vi "amplitude Spectrum from DAQ cernox removed.vi"(11 "Sample Duration (sec)":u32(knob)=31 scale=1.0..33.0) -> ()   [LabVIEW 2010]
uses:
  <vilib>/Analysis/2dsp.llb/Complex FFT.vi
  <vilib>/Analysis/NI_AALPro.lvlib
panel:
  out "error out":errorcluster
  out "Numeric":dbl=1484646840.0
  out "size(s)":i32=257
  out "Temp (K)":dbl=285.2027629999985 format="%_5g"
  in  "?":u16(ring)=5 items=["2", "4", "8", "16", "32", "64", "128", "256", "512", "8192", "1024", "2048", "4096", "8192", "16384", "32768", "65536", "131072", "262144", "524288 (one Channel)"]
  out "Spring Constant":dbl=0.016711730050282706
  out "<X^2>":dbl=2.3562204125555914e-19
  in  "Vpp":dbl=2.0
  out "x/y":cdb[](array[numeric])=[1.822835740797244e-23+0.0i, 1.7675640290457217e-23+0.0i, 1.4131702570700112e-23+0.0i, 2.223228937284431e-23+0.0i, 1.8861746568658304e-23+0.0i, 1.7224162597684228e-23+0.0i, 1.9293974775985452e-23+0.0i, 1.7742568740748702e-23+0.0i, 1.7769988182972965e-23+0.0i, 1.696176827526328e-23+0.0i, 1.8264193162076468e-23+0.0i, 1.9320144282170158e-23+0.0i, 2.0438742275850636e-23+0.0i, 2.222965311780456e-23+0.0i, 2.2549713226001863e-23+0.0i, 1.768885151694379e-23+0.0i, 2.176124999620469e-23+0.0i, 2.129234808266423e-23+0.0i, 2.067533774251591e-23+0.0i, 2.8427194668312566e-23+0.0i, 4.7553300725519583e-23+0.0i, 7.584325194857353e-23+0.0i, 2.1639134957441051e-23+0.0i, 2.5848083814905796e-23+0.0i, 2.851360155046589e-23+0.0i, 2.800634573630391e-23+0.0i, 2.338011797798725e-23+0.0i, 1.765079942656028e-23+0.0i, 2.104025187275973e-23+0.0i, 2.388051905691794e-23+0.0i, 2.853642619630031e-23+0.0i, 2.6711089516925724e-23+0.0i, 3.0459849796946806e-23+0.0i, 2.4401708416353815e-23+0.0i, 2.680531554902485e-23+0.0i, 2.9187825564451e-23+0.0i, 2.757565093207759e-23+0.0i, 3.035983267786727e-23+0.0i, 3.0910445814793146e-23+0.0i, 2.6051056874131243e-23+0.0i, 3.3956681306471256e-23+0.0i, 1.440691698306415e-22+0.0i, 6.100033131698352e-23+0.0i, 4.785561997662565e-23+0.0i, 4.4124379844200306e-23+0.0i, 4.1259461883143996e-23+0.0i, 3.976691477576303e-23+0.0i, 3.3602145359711534e-23+0.0i, 4.0934370310497964e-23+0.0i, 3.5625122285956665e-23+0.0i, 4.741274194370224e-23+0.0i, 4.622208059213624e-23+0.0i, 3.9223525205613755e-23+0.0i, 5.48665968324749e-23+0.0i, 3.875217807549581e-23+0.0i, 4.7796852328905696e-23+0.0i, 4.186904482333236e-23+0.0i, 6.049046606211197e-23+0.0i, 4.7905740078949955e-23+0.0i, 5.966921181453847e-23+0.0i, 5.130685417892801e-23+0.0i, 6.447729060239504e-23+0.0i, 6.070995523877117e-23+0.0i, 6.695912635778031e-23+0.0i, 5.982200688789285e-23+0.0i, 6.953655879559275e-23+0.0i, 7.719151718181244e-23+0.0i, 6.283551098164771e-23+0.0i, 6.616623115972441e-23+0.0i, 7.596763060682753e-23+0.0i, 7.333888292538558e-23+0.0i, 8.555537111075796e-23+0.0i, 9.5817232840548e-23+0.0i, 1.3181714014662204e-22+0.0i, 9.157484291226144e-23+0.0i, 7.751487205370229e-23+0.0i, 9.705897696242533e-23+0.0i, 1.0223323442116599e-22+0.0i, 1.0459001593217017e-22+0.0i, 1.1453450352921381e-22+0.0i, 1.2931657458720736e-22+0.0i, 1.459314628472842e-22+0.0i, 1.4070158876888328e-22+0.0i, 1.2605113149888989e-22+0.0i, 1.509819076598123e-22+0.0i, 1.544803841468646e-22+0.0i, 1.7700865059628094e-22+0.0i, 1.5376972478878197e-22+0.0i, 1.774728514817178e-22+0.0i, 1.8428914385759788e-22+0.0i, 2.2701171686531848e-22+0.0i, 1.838974511711876e-22+0.0i, 2.3627238680060907e-22+0.0i, 2.6269788328421313e-22+0.0i, 3.1051675808314644e-22+0.0i, 3.1120553407649953e-22+0.0i, 2.474307852966178e-22+0.0i, 3.341689824691674e-22+0.0i, 3.4471645453619096e-22+0.0i, 3.893320019912561e-22+0.0i, 4.1555515373755697e-22+0.0i, 5.455595521720538e-22+0.0i, 4.19934391425876e-22+0.0i, 4.908920977628759e-22+0.0i, 6.54725607731936e-22+0.0i, 5.404398330184923e-22+0.0i, 5.070609745440634e-22+0.0i, 7.501899902695688e-22+0.0i, 7.690047558843619e-22+0.0i, 8.091732940709215e-22+0.0i, 1.3031158912345799e-21+0.0i, 1.1512072647056174e-21+0.0i, 1.5268653969019806e-21+0.0i, 1.2878353575945014e-21+0.0i, 1.5861964752201703e-21+0.0i, 2.0874276416653818e-21+0.0i, 2.1537295587433287e-21+0.0i, 2.609801356487359e-21+0.0i, 2.794904862045169e-21+0.0i, 4.450890917281775e-21+0.0i, 4.782323183717228e-21+0.0i, 7.332879493133011e-21+0.0i, 8.720096388166533e-21+0.0i, 1.2048295246993849e-20+0.0i, 1.2445896073270755e-20+0.0i, 1.621889890374649e-20+0.0i, 2.5789862100239256e-20+0.0i, 1.7162750008545038e-20+0.0i, 1.6981422368097548e-20+0.0i, 1.1590736557342194e-20+0.0i, 9.14433437194095e-21+0.0i, 8.479983483390395e-21+0.0i, 6.568566536262503e-21+0.0i, 5.68343630205877e-21+0.0i, 4.478108035357037e-21+0.0i, 3.3395244446396683e-21+0.0i, 2.7493880233410565e-21+0.0i, 2.8389909650442048e-21+0.0i, 2.10455365672315e-21+0.0i, 1.5813034454830923e-21+0.0i, 1.2930365806113183e-21+0.0i, 1.2472170782254345e-21+0.0i, 1.1031647973872676e-21+0.0i, 8.8935516799099e-22+0.0i, 8.813468505072157e-22+0.0i, 8.834919269545325e-22+0.0i, 7.189279924592954e-22+0.0i, 8.018325795498779e-22+0.0i, 6.887070160521788e-22+0.0i, 7.329693497748081e-22+0.0i, 1.0058798260443032e-21+0.0i, 9.647467233858385e-22+0.0i, 5.881439114977712e-22+0.0i, 4.749433371668375e-22+0.0i, 3.6445918034601733e-22+0.0i, 2.8553400941847603e-22+0.0i, 3.9590897313916664e-22+0.0i, 3.3470734663309492e-22+0.0i, 3.2677511578285326e-22+0.0i, 2.7568964497043927e-22+0.0i, 2.243714895267099e-22+0.0i, 2.3930849601002674e-22+0.0i, 2.1787404973653707e-22+0.0i, 2.564842365349928e-22+0.0i, 1.8072546820279964e-22+0.0i, 2.008643480727801e-22+0.0i, 2.0432481222384193e-22+0.0i, 1.5072645039398344e-22+0.0i, 1.1578159171670506e-22+0.0i, 1.3856476941890455e-22+0.0i, 1.5750834082476817e-22+0.0i, 1.6598137898047965e-22+0.0i, 1.6846717057439265e-22+0.0i, 1.0637472542076113e-22+0.0i, 1.204765852625695e-22+0.0i, 1.1192400535353832e-22+0.0i, 9.586293087531511e-23+0.0i, 1.05741985863128e-22+0.0i, 1.0756461776754148e-22+0.0i, 1.0633342834367033e-22+0.0i, 9.41450875281874e-23+0.0i, 9.796297730479969e-23+0.0i, 8.991253125127156e-23+0.0i, 7.21495012420243e-23+0.0i, 8.108566724947074e-23+0.0i, 8.065267752833244e-23+0.0i, 8.159100620339912e-23+0.0i, 6.537407040699658e-23+0.0i, 6.065196292025972e-23+0.0i, 6.912565683967239e-23+0.0i, 4.585047711312349e-23+0.0i, 5.407319623212663e-23+0.0i, 5.662637982484711e-23+0.0i, 6.826102675920094e-23+0.0i, 5.317752314345768e-23+0.0i, 6.080938507048622e-23+0.0i, 5.580121915088842e-23+0.0i, 5.08599202552338e-23+0.0i, 5.757992131668778e-23+0.0i, 5.06295037704728e-23+0.0i, 4.0664759451789855e-23+0.0i, 8.778521018866551e-23+0.0i, 7.277091477651407e-23+0.0i, 3.968581632591024e-23+0.0i, 4.7007347174208957e-23+0.0i, 3.794186298189703e-23+0.0i, 4.820976496823016e-23+0.0i, 3.601765577546427e-23+0.0i, 3.459047542602718e-23+0.0i, 2.922903524340481e-23+0.0i, 3.570082548445812e-23+0.0i, 4.2755954972988234e-23+0.0i, 6.38478352818444e-23+0.0i, 1.601945502273552e-22+0.0i, 4.1400733672163123e-23+0.0i, 3.208702560959063e-23+0.0i, 3.3199369569753925e-23+0.0i, 2.7585085524308984e-23+0.0i, 3.131294045384947e-23+0.0i, 3.132076096760791e-23+0.0i, 2.5044550632070505e-23+0.0i, 2.996800434607099e-23+0.0i, 2.603310734333486e-23+0.0i, 2.3624545316458745e-23+0.0i, 2.8416716343560486e-23+0.0i, 2.5713096089926784e-23+0.0i, 2.3991585444755748e-23+0.0i, 2.3758300262426874e-23+0.0i, 2.894242043071023e-23+0.0i, 3.0079952252920497e-23+0.0i, 2.687090320067224e-23+0.0i, 3.060055893657326e-23+0.0i, 2.588927969919409e-23+0.0i, 1.3050755525240973e-22+0.0i, 6.369169567192907e-23+0.0i, 2.768674461007611e-23+0.0i, 1.996611478830249e-23+0.0i, 2.2847349020279004e-23+0.0i, 2.178447279898464e-23+0.0i, 1.611552403721389e-23+0.0i, 2.238567254293866e-23+0.0i, 2.0453257588723553e-23+0.0i, 2.2271941970345648e-23+0.0i, 2.0056331268074712e-23+0.0i, 1.60966633920541e-23+0.0i, 1.6230214465249225e-23+0.0i, 2.0086198141015995e-23+0.0i, 2.011029187025087e-23+0.0i, 1.980316992576717e-23+0.0i, 1.882256216302402e-23+0.0i, 1.974131492412098e-23+0.0i, 2.326555234354055e-23+0.0i, 1.515444684592899e-23+0.0i, 1.6225332592048996e-23+0.0i, 1.8662819972339634e-23+0.0i, 2.3769145357012108e-23+0.0i]
  out "df (Hz)":dbl=0.125
  out "time intervals":dbl=4.0
  out "iterations":dbl=64.0
  in  "# of points to collect":u16(ring)=2 items=["64", "128", "256", "512", "1024", "2048", "4096", "8192", "16384", "32768", "65536", "131072", "262144", "524288"]
  out "Cycles":dbl=1.0
  in  "Averages":dbl=1.0
  out "Total  points":dbl=16384.0
  out "XY Graph 3":cluster{dbl, dbl}[](graph)=[{6354.705, 1.822835740797244e-23}, {6354.83, 1.7675640290457217e-23}, {6354.955, 1.4131702570700112e-23}, {6355.08, 2.223228937284431e-23}, {6355.205, 1.8861746568658304e-23}, {6355.33, 1.7224162597684228e-23}, {6355.455, 1.9293974775985452e-23}, {6355.58, 1.7742568740748702e-23}, {6355.705, 1.7769988182972965e-23}, {6355.83, 1.696176827526328e-23}, {6355.955, 1.8264193162076468e-23}, {6356.08, 1.9320144282170158e-23}, {6356.205, 2.0438742275850636e-23}, {6356.33, 2.222965311780456e-23}, {6356.455, 2.2549713226001863e-23}, {6356.58, 1.768885151694379e-23}, {6356.705, 2.176124999620469e-23}, {6356.83, 2.129234808266423e-23}, {6356.955, 2.067533774251591e-23}, {6357.08, 2.8427194668312566e-23}, {6357.205, 4.7553300725519583e-23}, {6357.33, 7.584325194857353e-23}, {6357.455, 2.1639134957441051e-23}, {6357.58, 2.5848083814905796e-23}, {6357.705, 2.851360155046589e-23}, {6357.83, 2.800634573630391e-23}, {6357.955, 2.338011797798725e-23}, {6358.08, 1.765079942656028e-23}, {6358.205, 2.104025187275973e-23}, {6358.33, 2.388051905691794e-23}, {6358.455, 2.853642619630031e-23}, {6358.58, 2.6711089516925724e-23}, {6358.705, 3.0459849796946806e-23}, {6358.83, 2.4401708416353815e-23}, {6358.955, 2.680531554902485e-23}, {6359.08, 2.9187825564451e-23}, {6359.205, 2.757565093207759e-23}, {6359.33, 3.035983267786727e-23}, {6359.455, 3.0910445814793146e-23}, {6359.58, 2.6051056874131243e-23}, {6359.705, 3.3956681306471256e-23}, {6359.83, 1.440691698306415e-22}, {6359.955, 6.100033131698352e-23}, {6360.08, 4.785561997662565e-23}, {6360.205, 4.4124379844200306e-23}, {6360.33, 4.1259461883143996e-23}, {6360.455, 3.976691477576303e-23}, {6360.58, 3.3602145359711534e-23}, {6360.705, 4.0934370310497964e-23}, {6360.83, 3.5625122285956665e-23}, {6360.955, 4.741274194370224e-23}, {6361.08, 4.622208059213624e-23}, {6361.205, 3.9223525205613755e-23}, {6361.33, 5.48665968324749e-23}, {6361.455, 3.875217807549581e-23}, {6361.58, 4.7796852328905696e-23}, {6361.705, 4.186904482333236e-23}, {6361.83, 6.049046606211197e-23}, {6361.955, 4.7905740078949955e-23}, {6362.08, 5.966921181453847e-23}, {6362.205, 5.130685417892801e-23}, {6362.33, 6.447729060239504e-23}, {6362.455, 6.070995523877117e-23}, {6362.58, 6.695912635778031e-23}, {6362.705, 5.982200688789285e-23}, {6362.83, 6.953655879559275e-23}, {6362.955, 7.719151718181244e-23}, {6363.08, 6.283551098164771e-23}, {6363.205, 6.616623115972441e-23}, {6363.33, 7.596763060682753e-23}, {6363.455, 7.333888292538558e-23}, {6363.58, 8.555537111075796e-23}, {6363.705, 9.5817232840548e-23}, {6363.83, 1.3181714014662204e-22}, {6363.955, 9.157484291226144e-23}, {6364.08, 7.751487205370229e-23}, {6364.205, 9.705897696242533e-23}, {6364.33, 1.0223323442116599e-22}, {6364.455, 1.0459001593217017e-22}, {6364.58, 1.1453450352921381e-22}, {6364.705, 1.2931657458720736e-22}, {6364.83, 1.459314628472842e-22}, {6364.955, 1.4070158876888328e-22}, {6365.08, 1.2605113149888989e-22}, {6365.205, 1.509819076598123e-22}, {6365.33, 1.544803841468646e-22}, {6365.455, 1.7700865059628094e-22}, {6365.58, 1.5376972478878197e-22}, {6365.705, 1.774728514817178e-22}, {6365.83, 1.8428914385759788e-22}, {6365.955, 2.2701171686531848e-22}, {6366.08, 1.838974511711876e-22}, {6366.205, 2.3627238680060907e-22}, {6366.33, 2.6269788328421313e-22}, {6366.455, 3.1051675808314644e-22}, {6366.58, 3.1120553407649953e-22}, {6366.705, 2.474307852966178e-22}, {6366.83, 3.341689824691674e-22}, {6366.955, 3.4471645453619096e-22}, {6367.08, 3.893320019912561e-22}, {6367.205, 4.1555515373755697e-22}, {6367.33, 5.455595521720538e-22}, {6367.455, 4.19934391425876e-22}, {6367.58, 4.908920977628759e-22}, {6367.705, 6.54725607731936e-22}, {6367.83, 5.404398330184923e-22}, {6367.955, 5.070609745440634e-22}, {6368.08, 7.501899902695688e-22}, {6368.205, 7.690047558843619e-22}, {6368.33, 8.091732940709215e-22}, {6368.455, 1.3031158912345799e-21}, {6368.58, 1.1512072647056174e-21}, {6368.705, 1.5268653969019806e-21}, {6368.83, 1.2878353575945014e-21}, {6368.955, 1.5861964752201703e-21}, {6369.08, 2.0874276416653818e-21}, {6369.205, 2.1537295587433287e-21}, {6369.33, 2.609801356487359e-21}, {6369.455, 2.794904862045169e-21}, {6369.58, 4.450890917281775e-21}, {6369.705, 4.782323183717228e-21}, {6369.83, 7.332879493133011e-21}, {6369.955, 8.720096388166533e-21}, {6370.08, 1.2048295246993849e-20}, {6370.205, 1.2445896073270755e-20}, {6370.33, 1.621889890374649e-20}, {6370.455, 2.5789862100239256e-20}, {6370.58, 1.7162750008545038e-20}, {6370.705, 1.6981422368097548e-20}, {6370.83, 1.1590736557342194e-20}, {6370.955, 9.14433437194095e-21}, {6371.08, 8.479983483390395e-21}, {6371.205, 6.568566536262503e-21}, {6371.33, 5.68343630205877e-21}, {6371.455, 4.478108035357037e-21}, {6371.58, 3.3395244446396683e-21}, {6371.705, 2.7493880233410565e-21}, {6371.83, 2.8389909650442048e-21}, {6371.955, 2.10455365672315e-21}, {6372.08, 1.5813034454830923e-21}, {6372.205, 1.2930365806113183e-21}, {6372.33, 1.2472170782254345e-21}, {6372.455, 1.1031647973872676e-21}, {6372.58, 8.8935516799099e-22}, {6372.705, 8.813468505072157e-22}, {6372.83, 8.834919269545325e-22}, {6372.955, 7.189279924592954e-22}, {6373.08, 8.018325795498779e-22}, {6373.205, 6.887070160521788e-22}, {6373.33, 7.329693497748081e-22}, {6373.455, 1.0058798260443032e-21}, {6373.58, 9.647467233858385e-22}, {6373.705, 5.881439114977712e-22}, {6373.83, 4.749433371668375e-22}, {6373.955, 3.6445918034601733e-22}, {6374.08, 2.8553400941847603e-22}, {6374.205, 3.9590897313916664e-22}, {6374.33, 3.3470734663309492e-22}, {6374.455, 3.2677511578285326e-22}, {6374.58, 2.7568964497043927e-22}, {6374.705, 2.243714895267099e-22}, {6374.83, 2.3930849601002674e-22}, {6374.955, 2.1787404973653707e-22}, {6375.08, 2.564842365349928e-22}, {6375.205, 1.8072546820279964e-22}, {6375.33, 2.008643480727801e-22}, {6375.455, 2.0432481222384193e-22}, {6375.58, 1.5072645039398344e-22}, {6375.705, 1.1578159171670506e-22}, {6375.83, 1.3856476941890455e-22}, {6375.955, 1.5750834082476817e-22}, {6376.08, 1.6598137898047965e-22}, {6376.205, 1.6846717057439265e-22}, {6376.33, 1.0637472542076113e-22}, {6376.455, 1.204765852625695e-22}, {6376.58, 1.1192400535353832e-22}, {6376.705, 9.586293087531511e-23}, {6376.83, 1.05741985863128e-22}, {6376.955, 1.0756461776754148e-22}, {6377.08, 1.0633342834367033e-22}, {6377.205, 9.41450875281874e-23}, {6377.33, 9.796297730479969e-23}, {6377.455, 8.991253125127156e-23}, {6377.58, 7.21495012420243e-23}, {6377.705, 8.108566724947074e-23}, {6377.83, 8.065267752833244e-23}, {6377.955, 8.159100620339912e-23}, {6378.08, 6.537407040699658e-23}, {6378.205, 6.065196292025972e-23}, {6378.33, 6.912565683967239e-23}, {6378.455, 4.585047711312349e-23}, {6378.58, 5.407319623212663e-23}, {6378.705, 5.662637982484711e-23}, {6378.83, 6.826102675920094e-23}, {6378.955, 5.317752314345768e-23}, {6379.08, 6.080938507048622e-23}, {6379.205, 5.580121915088842e-23}, {6379.33, 5.08599202552338e-23}, {6379.455, 5.757992131668778e-23}, {6379.58, 5.06295037704728e-23}, {6379.705, 4.0664759451789855e-23}, {6379.83, 8.778521018866551e-23}, {6379.955, 7.277091477651407e-23}, {6380.08, 3.968581632591024e-23}, {6380.205, 4.7007347174208957e-23}, {6380.33, 3.794186298189703e-23}, {6380.455, 4.820976496823016e-23}, {6380.58, 3.601765577546427e-23}, {6380.705, 3.459047542602718e-23}, {6380.83, 2.922903524340481e-23}, {6380.955, 3.570082548445812e-23}, {6381.08, 4.2755954972988234e-23}, {6381.205, 6.38478352818444e-23}, {6381.33, 1.601945502273552e-22}, {6381.455, 4.1400733672163123e-23}, {6381.58, 3.208702560959063e-23}, {6381.705, 3.3199369569753925e-23}, {6381.83, 2.7585085524308984e-23}, {6381.955, 3.131294045384947e-23}, {6382.08, 3.132076096760791e-23}, {6382.205, 2.5044550632070505e-23}, {6382.33, 2.996800434607099e-23}, {6382.455, 2.603310734333486e-23}, {6382.58, 2.3624545316458745e-23}, {6382.705, 2.8416716343560486e-23}, {6382.83, 2.5713096089926784e-23}, {6382.955, 2.3991585444755748e-23}, {6383.08, 2.3758300262426874e-23}, {6383.205, 2.894242043071023e-23}, {6383.33, 3.0079952252920497e-23}, {6383.455, 2.687090320067224e-23}, {6383.58, 3.060055893657326e-23}, {6383.705, 2.588927969919409e-23}, {6383.83, 1.3050755525240973e-22}, {6383.955, 6.369169567192907e-23}, {6384.08, 2.768674461007611e-23}, {6384.205, 1.996611478830249e-23}, {6384.33, 2.2847349020279004e-23}, {6384.455, 2.178447279898464e-23}, {6384.58, 1.611552403721389e-23}, {6384.705, 2.238567254293866e-23}, {6384.83, 2.0453257588723553e-23}, {6384.955, 2.2271941970345648e-23}, {6385.08, 2.0056331268074712e-23}, {6385.205, 1.60966633920541e-23}, {6385.33, 1.6230214465249225e-23}, {6385.455, 2.0086198141015995e-23}, {6385.58, 2.011029187025087e-23}, {6385.705, 1.980316992576717e-23}, {6385.83, 1.882256216302402e-23}, {6385.955, 1.974131492412098e-23}, {6386.08, 2.326555234354055e-23}, {6386.205, 1.515444684592899e-23}, {6386.33, 1.6225332592048996e-23}, {6386.455, 1.8662819972339634e-23}, {6386.58, 2.3769145357012108e-23}]
  out "freq range (hz)":dbl=32.0
  out "dt (s)":dbl=0.015625
  in  "Sensitivity":u16(ring)=22 items=["2 nV/fA", "5 nV/fA", "10 nV/fA", "20 nV/fA", "50 nV/fA", "100 nV/fA", "200 nV/fA", "500 nV/fA", "1 uV/pA", "2 uV/pA", "5 uV/pA", "10 uV/pA", "20 uV/pA", "50 uV/pA", "100 uV/pA", "200 uV/pA", "500 uV/pA", "1 mV/nA", "2 mV/nA", "5 mV/nA", "10 mV/nA", "20 mV/nA", "50 mV/nA", "100 mV/nA", "200 mV/nA", "500 mV/nA", "1 V/uA"]
  in  "Data to Store":u16(ring) items=["X and Y", "R and Theta"]
  in  "Sampling Rate":u16(ring)=13 items=["62.5 mHz", "125 mHz", "250 mHz", "500 mHz", "1 Hz", "2 Hz", "4 Hz", "8 Hz", "16 Hz", "32 Hz", "64 Hz, 256 s wait", "128 Hz, 128 s wait", "256 Hz, 64 s wait", "512 Hz, 32 s wait"]
  in  "Center Frequency [Hz]":dbl=6370.58 format="%.3f"
  in  "Detection Bandwidth":u16(ring)=5 items=["25 kHz", "8.33 kHz", "2.50 kHz", "833 Hz", "250 Hz", "83.3 Hz", "25 Hz", "8.33 Hz", "2.50 Hz", "0.833 Hz", "0.250 Hz", "0.0833 Hz", "0.025 Hz"]
  in  "DS 345 GPIB Address":i32=19
  in  "SR 830 GPIB Address":i32=8
  # "Bandwidth>\n2*samp rate"
  # "SR 830"
  # "Adquisition DAQ"
  # "Sample Rate DAQ"
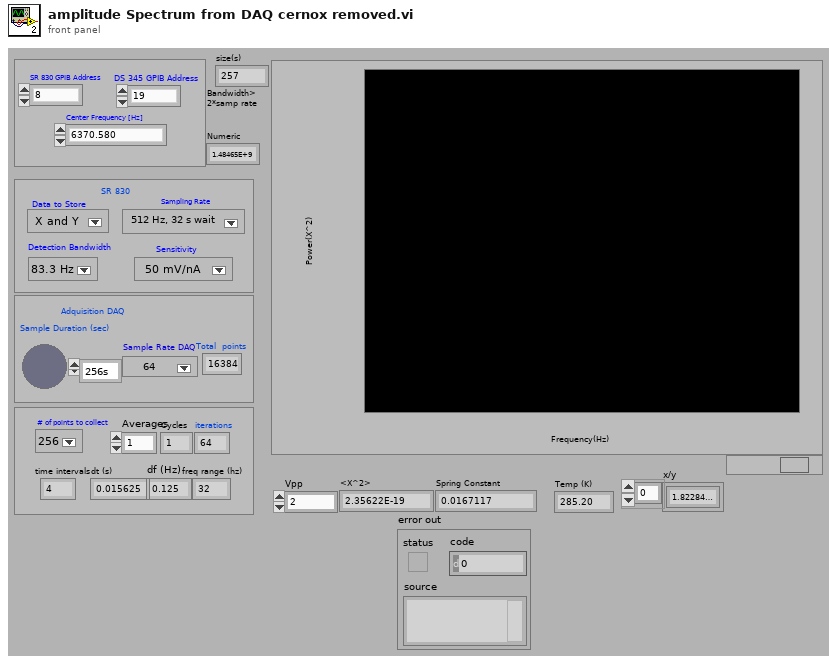
[diagram p1: front panel]
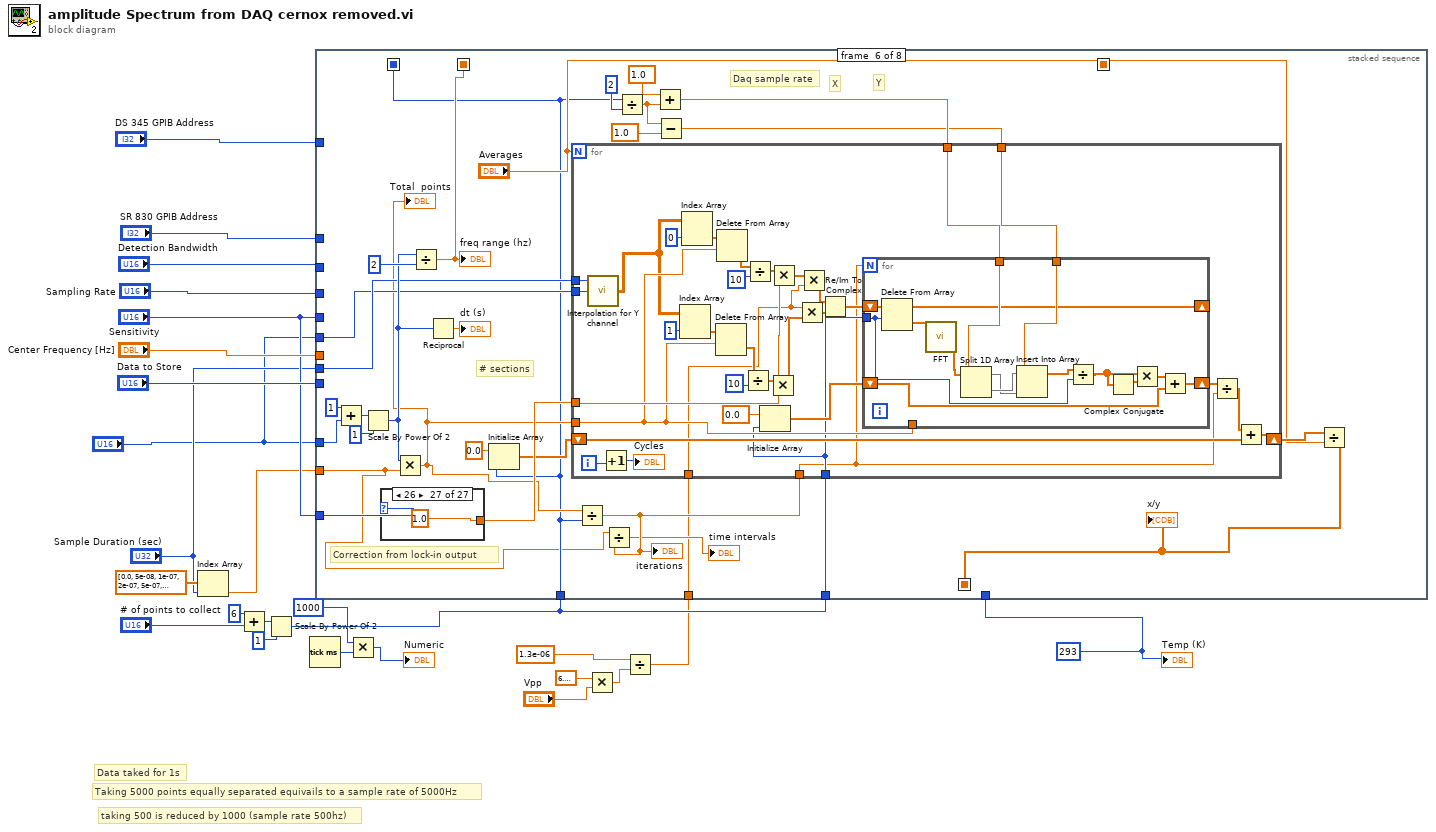
[diagram p0: block diagram]
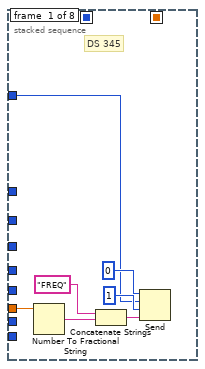
[diagram p2: hidden frame]
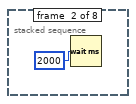
[diagram p3: hidden frame]
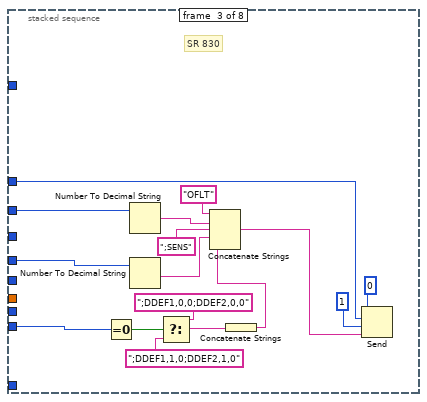
[diagram p4: hidden frame]
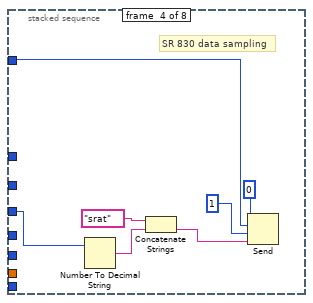
[diagram p5: hidden frame]
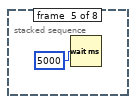
[diagram p6: hidden frame]
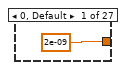
[diagram p7: hidden frame]
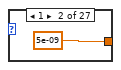
[diagram p8: hidden frame]
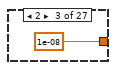
[diagram p9: hidden frame]
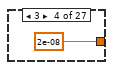
[diagram p10: hidden frame]
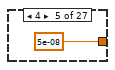
[diagram p11: hidden frame]
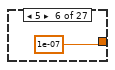
[diagram p12: hidden frame]
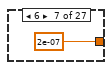
[diagram p13: hidden frame]
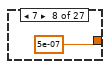
[diagram p14: hidden frame]
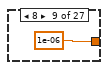
[diagram p15: hidden frame]
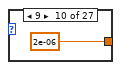
[diagram p16: hidden frame]
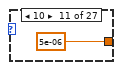
[diagram p17: hidden frame]
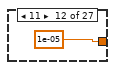
[diagram p18: hidden frame]
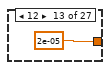
[diagram p19: hidden frame]
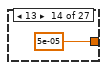
[diagram p20: hidden frame]
diagram:
  w1 = 293
  # "taking 500 is reduced by 1000 (sample rate 500hz)"
  # "Data taked for 1s"
  # "Taking 5000 points equally separated equivails to a sample rate of 5000Hz"
  n1 = Index Array(array=dbl[] [0.0, 5e-08, 1e-07, 2e-07, 5e-07, 1e-06, 2e-06, 5e-06, 1e-05, 2e-05, 5e-05, 0.0001, 0.0002, 0.0005, 0.001, 0.002, 0.005, 0.01, 0.02, 0.05, 0.1, 0.2, 0.5, 1.0, 2.0, 5.0, 10.0, 16.0, 32.0, 64.0, 128.0, 256.0, 512.0, 1024.0], index="Sample Duration (sec)") -> (element=w17:dbl)
  n2 = Add(x=6, y="# of points to collect") -> (x+y=w13:i32)
  n3 = Scale By Power Of 2(n=w13, x=1) -> (x*2^n=w11:i32)
  n4 = Tick Count (ms)() -> (millisecond timer value=w4:u32)
  n5 = Multiply(x=1000, y=w4) -> (x*y=→"Numeric":u32)
  n6 = Multiply(x=6.283185307179586, y="Vpp") -> (x*y=w8:dbl)
  n7 = Divide(x=1.3e-06 ("wave Length"), y=w8) -> (x/y=w6:dbl)
  n8 = stacked-sequence {
    seq-local: [_ _ _ _ _ w62 _ _] -> [_ _ _ _ _ _ w180 _]
    seq-local: [_ _ _ _ _ w81 _ _] -> [_ _ _ _ _ _ w178 _]
    seq-local: [_ _ _ _ _ w69 _ _] -> [_ _ _ _ _ _ w176 _]
    seq-local: [_ _ _ _ _ _ w169 _] -> [_ _ _ _ _ _ _ _]
    tunnel: "Center Frequency [Hz]" -> [w27 _ _ _ _ _ w188 _]
    tunnel: "DS 345 GPIB Address" -> [w26 _ _ w51 _ _ _ _]
    tunnel: "SR 830 GPIB Address" -> [_ _ w37 _ _ _ _ _]
    tunnel: "Detection Bandwidth" -> [_ _ w36 _ _ _ _ _]
    tunnel: "Sensitivity" -> [_ _ w35 _ _ _ _ _]
    tunnel: "Data to Store" -> [_ _ w34 _ _ _ _ _]
    tunnel: "Sampling Rate" -> [_ _ _ w50 _ _ _ _]
    tunnel: "?" -> [_ _ _ _ _ w84 _ _]
    tunnel: "Sensitivity" -> [_ _ _ _ _ w80 _ _]
    tunnel: w17 -> [_ _ _ _ _ w61 _ _]
    tunnel: "Sample Duration (sec)" -> [_ _ _ _ _ w67 _ _]
    tunnel: "?" -> [_ _ _ _ _ w66 _ _]
    tunnel: w11 -> [_ _ _ _ _ w64 _ _]
    tunnel: w11 -> [_ _ _ _ _ w62 _ _]
    tunnel: w6 -> [_ _ _ _ _ w58 _ _]
    tunnel: w1 -> [_ _ _ _ _ _ w170 _]
    frame #0 {
      # "DS 345"
      n9 = Number To Fractional String(number=w27) -> (F-format string=w31:string)  [unwired: 3 out]
      n10 = Concatenate Strings("FREQ", w31) -> (w30:string)
      n11 = Send(0:0 ("bus"), 2:w26, 3:i16 1 ("mode"), 5:w30) -> ()  [unwired: 1 in, 3 out]
    }
    frame #1 {
      n12 = Wait (ms)(milliseconds to wait=2000) -> ()  [unwired: 1 out]
    }
    frame #2 {
      # "SR 830"
      n13 = Equal To 0?(x=w34) -> (x = 0?=w42:bool)
      n14 = Number To Decimal String(number=w36) -> (decimal integer string=w48:string)  [unwired: 1 out]
      n15 = Number To Decimal String(number=w35) -> (decimal integer string=w46:string)  [unwired: 1 out]
      n16 = Select(t=";DDEF1,0,0;DDEF2,0,0", s=w42, f=";DDEF1,1,0;DDEF2,1,0") -> (s? t:f=w41:string)
      n17 = Concatenate Strings(w41) -> (w40:string)
      n18 = Concatenate Strings("OFLT", w48, ";SENS", w46, w40) -> (w45:string)
      n19 = Send(0:0 ("bus"), 2:w37, 3:i16 1 ("mode"), 5:w45) -> ()  [unwired: 1 in, 3 out]
    }
    frame #3 {
      # "SR 830 data sampling"
      n20 = Number To Decimal String(number=w50) -> (decimal integer string=w55:string)  [unwired: 1 out]
      n21 = Concatenate Strings("srat", w55) -> (w54:string)
      n22 = Send(0:0 ("bus"), 2:w51, 3:i16 1 ("mode"), 5:w54) -> ()  [unwired: 1 in, 3 out]
    }
    frame #4 {
      n23 = Wait (ms)(milliseconds to wait=5000) -> ()  [unwired: 1 out]
    }
    frame #5 {
      # "Correction from lock-in output"
      # "Y"
      # "X"
      # "# sections"
      # "Daq sample rate"
      n24 = Add(x=1, y=w84) -> (x+y=w85:i32)
      n25 = Scale By Power Of 2(n=w85, x=1) -> (x*2^n=w68:i32)
      n26 = case shown="26" w80 {
        tunnel: [2e-09 5e-09 1e-08 2e-08 5e-08 1e-07 2e-07 5e-07 1e-06 2e-06 5e-06 1e-05 2e-05 5e-05 0.0001 0.0002 0.0005 0.001 0.002 0.005 0.01 0.02 0.05 0.1 0.2 0.5 1.0] -> w79
        frame 0, Default {
        }
        frame 1 {
        }
        frame 2 {
        }
        frame 3 {
        }
        frame 4 {
        }
        frame 5 {
        }
        frame 6 {
        }
        frame 7 {
        }
        frame 8 {
        }
        frame 9 {
        }
        frame 10 {
        }
        frame 11 {
        }
        frame 12 {
        }
        frame 13 {
        }
        frame 14 {
        }
        frame 15 {
        }
        frame 16 {
        }
        frame 17 {
        }
        frame 18 {
        }
        frame 19 {
        }
        frame 20 {
        }
        frame 21 {
        }
        frame 22 {
        }
        frame 23 {
        }
        frame 24 {
        }
        frame 25 {
        }
        frame 26 {
        }
      }
      n27 = Multiply(x=w68, y=w61) -> (x*y=w63:dbl)
      "Total  points" <- w63
      n28 = Divide(x=w68, y=2) -> (x/y=w81:dbl)
      "freq range (hz)" <- w81
      n29 = Reciprocal(x=w68) -> (1/x=→"dt (s)":dbl)
      n30 = Initialize Array(0.0, w62) -> (w65:dbl[])
      n31 = Divide(x=w63, y=w62) -> (x/y=w60:dbl)
      "iterations" <- w60
      n32 = Divide(x=w61, y=w60) -> (x/y=→"time intervals":dbl)
      n33 = Divide(x=w62, y=2) -> (x/y=w75:dbl)
      n34 = Add(x=1.0, y=w75) -> (x+y=w73:dbl)
      n35 = Subtract(x=w75, y=1.0) -> (x-y=w72:dbl)
      n36 = for {
        N: "Averages" -> [_]
        tunnel: w79 -> [w120]
        tunnel: w63 -> [w107]
        tunnel: w73 -> [w109]
        tunnel: w72 -> [w108]
        shift-right: [w105] -> w71
        shift-left: w65 -> [w106]
        tunnel: w67 -> [w104]
        tunnel: w66 -> [w88]
        tunnel: w64 -> [w98]
        tunnel: w60 -> [w97]
        tunnel: w58 -> [w89]
        i -> [w103]
        n37 = call "Interpolation for Y channel.vi"(2:w88, "Sample Duration (sec)"=w104) -> ("array w/ subset deleted"=w94:dbl[][])  [unwired: 1 out]
        n38 = Increment(x=w103) -> (x+1=→"Cycles":i32)
        n39 = Index Array(array=w94, index (row)=1) -> (element=w112:dbl[])  [unwired: 1 in]
        n40 = Index Array(array=w94, index (row)=0) -> (element=w113:dbl[])  [unwired: 1 in]
        n41 = Delete From Array(array=w112, length=w107) -> (deleted portion=w111:dbl[])  [unwired: 1 in, 1 out]
        n42 = Delete From Array(array=w113, length=w107) -> (deleted portion=w110:dbl[])  [unwired: 1 in, 1 out]
        n43 = Divide(x=w111, y=10) -> (x/y=w118:dbl[])
        n44 = Divide(x=w110, y=10) -> (x/y=w116:dbl[])
        n45 = Initialize Array(0.0 ("element"), w98) -> (w99:dbl[])
        n46 = Multiply(x=w118, y=w120) -> (x*y=w91:dbl[])
        n47 = Multiply(x=w116, y=w120) -> (x*y=w93:dbl[])
        n48 = Multiply(x=w89, y=w91) -> (x*y=w90:dbl[])
        n49 = Multiply(x=w93, y=w89) -> (x*y=w92:dbl[])
        n50 = Re/Im To Complex(1:w90, 2:w92) -> (0:w101:cdb[])
        n51 = for {
          N: w97 -> [_]
          tunnel: w109 -> [w135]
          tunnel: w108 -> [w134]
          tunnel: w107 -> [_]
          tunnel: w98 -> [w121]
          shift-right: [w129] -> _
          shift-left: w101 -> [w131]
          shift-right: [w126] -> w96
          shift-left: w99 -> [w125]
          n52 = Delete From Array(array=w131, length=w121) -> (deleted portion=w130:cdb[], array with subset deleted=w129:cdb[])  [unwired: 1 in]
          n53 = call-poly <vilib>:"FFT.vi"("X"=w130) -> ("FFT {X}"=w124:cdb[])  [unwired: 2 in, 8 out]
          n54 = Split 1D Array(array=w124, index=w135) -> (first subarray=w132:cdb[], second subarray=w133:cdb[])
          n55 = Insert Into Array(array=w133, index=w134, new element=w132) -> (w122:cdb[])
          n56 = Divide(x=w122, y=w121) -> (x/y=w123:cdb[])
          n57 = Complex Conjugate(1:w123) -> (0:w128:cdb[])
          n58 = Multiply(x=w123, y=w128) -> (x*y=w127:cdb[])
          n59 = Add(x=w127, y=w125) -> (x+y=w126:cdb[])
        }
        n60 = Divide(x=w96, y=w97) -> (x/y=w95:cdb[])
        n61 = Add(x=w95, y=w106) -> (x+y=w105:cdb[])
      }
      n62 = Divide(x=w71, y="Averages") -> (x/y=w69:cdb[])
      "x/y" <- w69
    }
    frame #6 {
      n63 = Divide(x=w178, y=2) -> (x/y=w187:dbl)
      n64 = Subtract(x=w188, y=w187) -> (x-y=w183:dbl)
      n65 = Initialize Array(w183, 1 ("dimension size")) -> (w184:dbl[])
      n66 = Array Size(array=w176) -> (size(s)=w179:i32)
      n67 = Divide(x=w178, y=w179) -> (x/y=w177:dbl)
      "df (Hz)" <- w177
      n68 = for {
        N: w180 -> [w204]
        shift-right: [w190] -> _
        shift-left: w183 -> [w206]
        tunnel: w177 -> [w205]
        shift-right: [w199] -> _
        shift-left: w176 -> [w202]
        shift-right: [w191] -> w165
        shift-left: w184 -> [w192]
        tunnel: [w190] -> w169 mode=indexing
        i -> [w194]
        n69 = Delete From Array(array=w202, length=1, index=0) -> (deleted portion=w198:cdb[], array with subset deleted=w199:cdb[])
        n70 = Add(x=1, y=w194) -> (x+y=w193:i32)
        n71 = Index Array(array=w198, index=0) -> (element=w189:cdb)
        n72 = Add(x=w206, y=w205) -> (x+y=w190:dbl)
        n73 = Insert Into Array(array=w192, index=w193, new element=w190) -> (w191:dbl[])
        n74 = Bundle(w190, w189) -> (w203:cluster{dbl, cdb})  [unwired: 1 out]
        n75 = call "XY Chart Buffer.vi"("chart length (points)"=w204, "new point"=w203) -> ("XY chart data"=→"XY Graph 3":cluster{"x":dbl, "y":dbl}[])  [unwired: 2 in, 7 out]
      }
      n76 = Array Size(array=w165) -> (size(s)=→"size(s)":i32)
      n77 = Interleave 1D Arrays(w165, w176) -> (w182:cdb[])
      n78 = Reshape Array(w182, w180, 2 ("dimension size")) -> (w168:cdb[][])
      n79 = Transpose 2D Array(2D array=w168) -> (transposed array=w166:cdb[][])
      n80 = call "Convert to Dynamic Data2"("2D Array"=w166) -> ("Dynamic Data Type"=w167:dynamicdata)  [unwired: 3 out]
      n81 = call "Write"("Signals"=w167) -> ()  [unwired: 6 in, 13 out]
      n82 = call "Convert to Dynamic Data"("Array"=w176) -> ("Dynamic Data Type"=w175:dynamicdata)  [unwired: 3 out]
      n83 = call "Integral (Sum[Xdt])"("Signals"=w175) -> ("error out"=→"error out":errorcluster, "Result"=w172:dynamicdata)  [unwired: 1 in, 4 out]
      "<X^2>" <- w172
      n84 = Multiply(x=1.38065e-23, y=w170) -> (x*y=w173:dbl)
      n85 = Divide(x=w173, y=w172) -> (x/y=→"Spring Constant":dynamicdata)
    }
    frame #7 {
    }
  }
  "Temp (K)" <- w1
